vi "S2C_XML_ManageResult.vi"(5 "LastTest?":bool, 7 "LastMeas?":bool, 8 "Error In":errorcluster, 11 "Result":T1) -> (0 "Error Out":errorcluster)   [LabVIEW 2015]
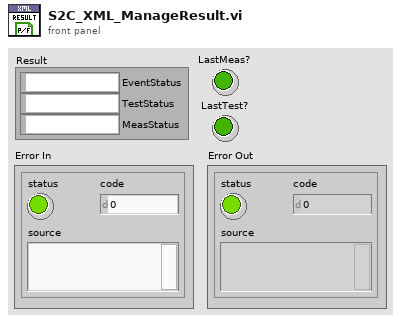
[diagram p1: front panel]
types:
  T1 = cluster{"EventStatus":string, "TestStatus":string, "MeasStatus":string}
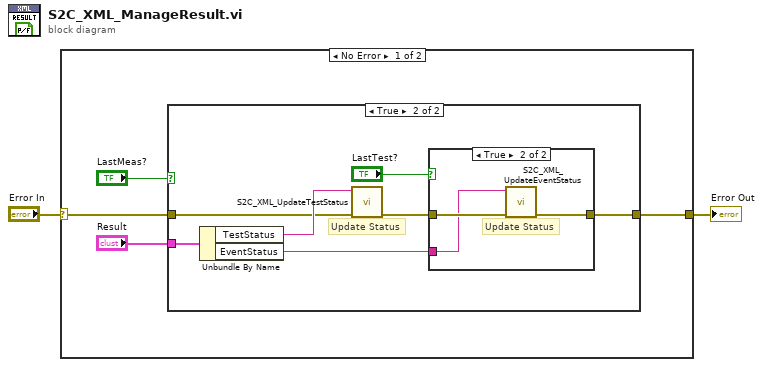
[diagram p0: block diagram]
diagram:
  n1 = case shown="No Error" "Error In" {
    selector: "Error In" -> [w5 w19]
    tunnel: [w3 w19] -> w1
    frame No Error {
      n2 = case shown="True" "LastMeas?" {
        tunnel: w5 -> [w7 w8]
        tunnel: "Result" -> [_ w14]
        tunnel: [w7 w11] -> w3
        frame False {
        }
        frame True {
          # "Update Status"
          n3 = Unbundle By Name(w14) -> ("TestStatus"=w9:string, "EventStatus"=w12:string)
          n4 = call "S2C_XML_UpdateTestStatus.vi"("Error In"=w8, "Result"=w9) -> ("Error Out"=w13:errorcluster)  [unwired: 9 in]
          n5 = case shown="True" "LastTest?" {
            tunnel: w13 -> [w15 w17]
            tunnel: w12 -> [_ w16]
            tunnel: [w15 w18] -> w11
            frame False {
            }
            frame True {
              # "Update Status"
              n6 = call "S2C_XML_UpdateEventStatus.vi"("Error In"=w17, "Value"=w16) -> ("Error Out"=w18:errorcluster)  [unwired: 9 in]
            }
          }
        }
      }
    }
    frame Error {
    }
  }
  "Error Out" <- w1
